vi "FPGA_bubble_SCTL_FIFO.vi"() -> ()   [LabVIEW 2020]
uses:
  <vilib>/Platform/TimedLoop/XDataNode/timing_clust.ctl
  <vilib>/Platform/TimedLoop/XDataNode/nitl_modes.ctl
  <vilib>/Platform/TimedLoop/XDataNode/wakeup.ctl
  <vilib>/rvi/interface/RandomDataEmulation/niFpgaRandomDataHandleErrors.vi
  <vilib>/rvi/Emulation/niFpgaSctlEmulationGetInTimedLoop.vi
  <vilib>/rvi/Emulation/niFpgaEmulationReportErrorSimple.vi
  <vilib>/rvi/Emulation/niFpgaGetClockAttributes.vi
  <vilib>/rvi/Emulation/niFpgaCriticalErrorInLSC.vi
  <vilib>/rvi/DataTransferAndStorage/Container/XNode/niFpgaContainer.xnode
  <vilib>/rvi/interface/RandomDataEmulation/nirviRandomDataFpgaReadWriteTemplate.vi
  <vilib>/platform/TimedLoop/XDataNode/XDataNode.xnode
  <vilib>/Platform/TimedLoop/XDataNode/XDNodeRunTimeDep.lvlib
panel:
  out "sort time (us)":u32
  out "Timed Out? FIFO index":bool
  out "Timed Out? FIFO list":bool
  out "Timed Out FIFO In":bool
  out "Output Valid":bool
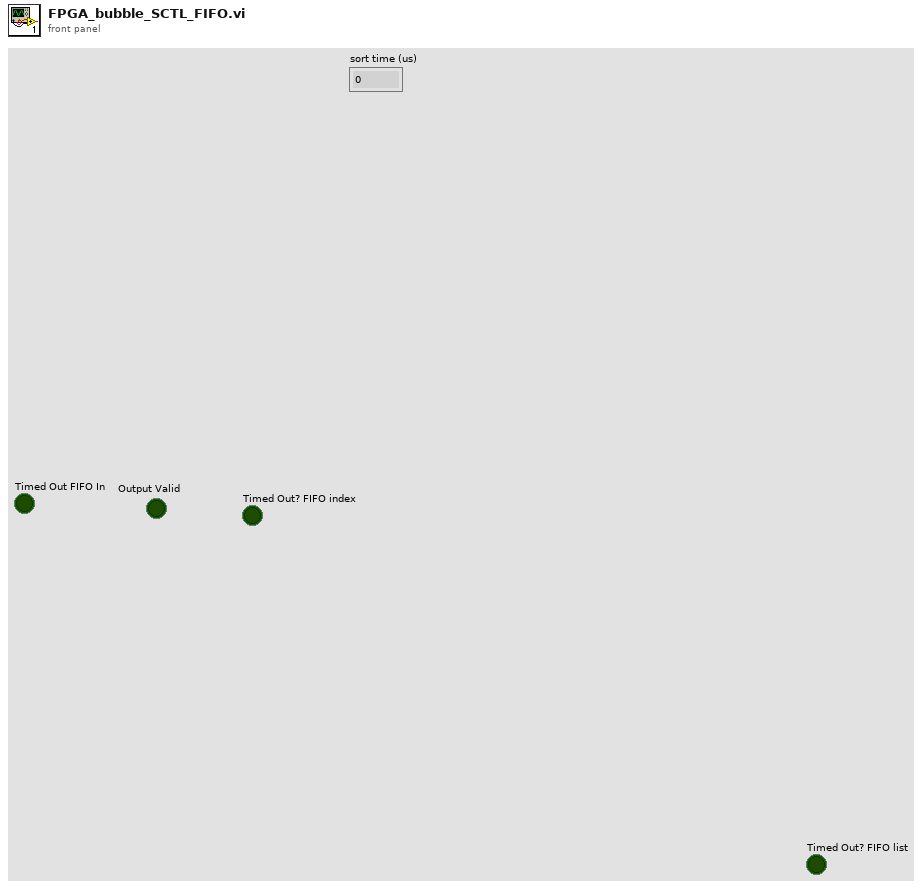
[diagram p1: front panel]
types:
  T1 = typedef "XDNodeRunTimeDep.lvlib/timing_clust.ctl" = cluster{"Expected End [f-1]":u64, "Actual End [f-1]":u64, "Finished Late? [f-1]":bool, "Expected End [i-1]":u64, "Actual End [i-1]":u64, "Finished Late? [i-1]":bool, "Expected Start [i]":u64, "Actual Start [i]":u64, "Expected Start [f]":u64, "Actual Start [f]":u64, "Source Name":string, "Structure Name":string, "Period":i64, "Deadline":i64, "Offset":i64, "Start":i64, "Priority":i32, "Timeout":i32, "Mode":T2, "Wakeup Reason":T3, "Error":errorcluster, "Source Type":string, "Secondary Source Type":string, "Global End Time":u64, "Global Start Time":u64, "Frame Duration":u64, "Iteration Duration":u64, "Assigned CPU":i32, "I/O Scan Engine Mode":u32}
  T2 = typedef "XDNodeRunTimeDep.lvlib/nitl_modes.ctl" = enum32{"No Change", "Process missed periods, maintain original phase", "Discard missed periods, maintain original phase", "Process missed periods, ignore original phase", "Discard missed periods, ignore original phase"}
  T3 = typedef "XDNodeRunTimeDep.lvlib/wakeup.ctl" = enum32{"Normal", "Aborted", "Asynchronous wakeup", "Timing source error", "Timed loop error", "Timeout"}
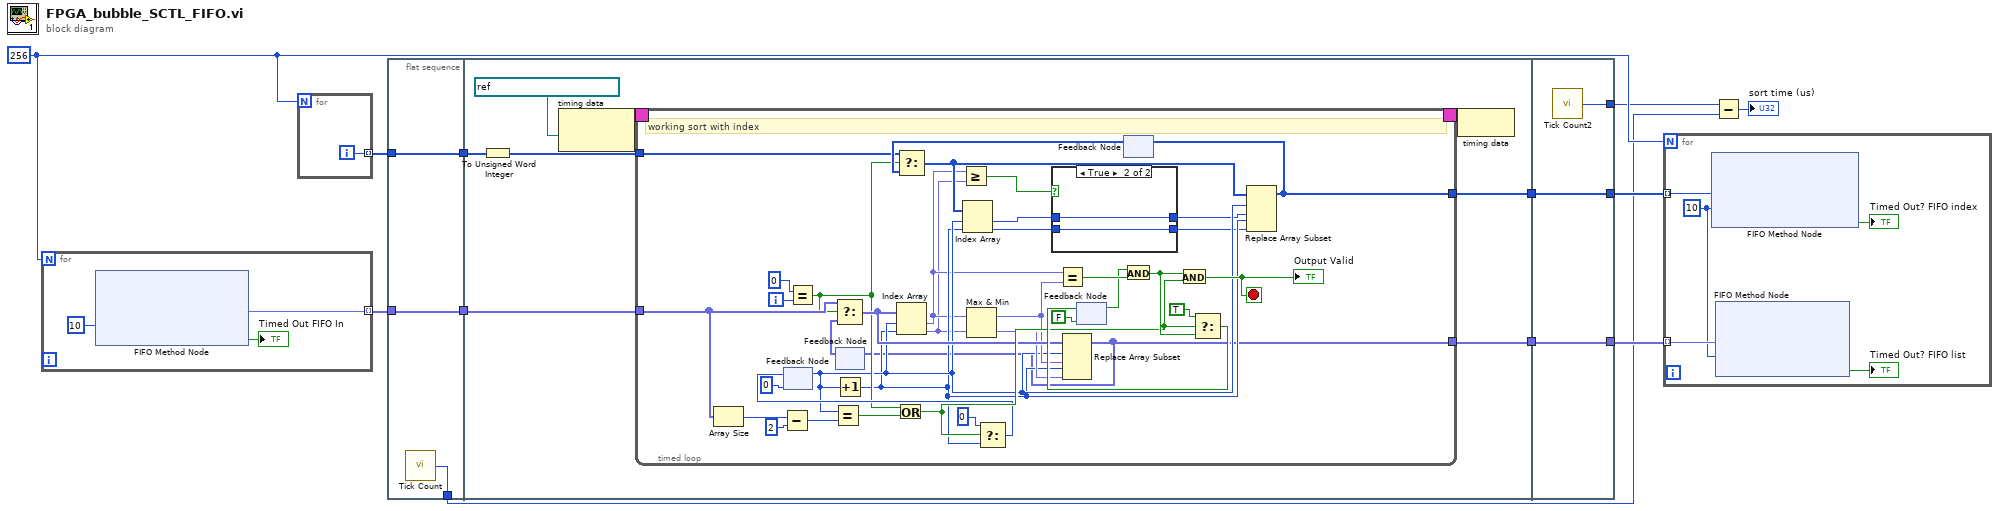
[diagram p0: block diagram]
diagram:
  w9 = 256
  n1 = for {
    N: w9 -> [_]
    tunnel: [w15] -> w11 mode=indexing
    n2 = xnode ("FIFO Method Node")("Timeout"=10) -> ("Element"=w15:fxp<+/-,16,4>, "Timed Out?"=→"Timed Out FIFO In":bool)  [unwired: 1 in, 1 out]
  }
  n3 = for {
    N: w9 -> [_]
    tunnel: [w16] -> w12 mode=indexing
    i -> [w16]
  }
  n4 = flat-sequence {
    tunnel: w11 -> [w18]
    tunnel: w12 -> [w19]
    tunnel: [w19] -> w7
    tunnel: [w18] -> w6
    tunnel: [w17] -> w2
    tunnel: w7 -> [w25]
    tunnel: w6 -> [w22]
    tunnel: [w21] -> w5
    tunnel: [w20] -> w4
    tunnel: [w76] -> w8
    tunnel: [w77] -> w10
    tunnel: w5 -> [w77]
    tunnel: w4 -> [w76]
    tunnel: [w75] -> w3
    frame #0 {
      n5 = call "Tick Count"() -> ("Tick Count(uSec)"=w17:u32)
    }
    frame #1 {
      n6 = To Unsigned Word Integer(number=w25) -> (unsigned 16bit integer=w24:u16[])
      n7 = node-c288(refnum<k21> "40 MHz Onboard Clock" ("Source Name")) -> (w27:T1)
      n8 = timed-loop {
        tunnel: w22 -> [w61]
        tunnel: w24 -> [w40]
        timing: w27 -> [_]
        timing-out: [_] -> w26
        tunnel: [w29] -> w21
        tunnel: [w28] -> w20
        i -> [w44]
        stop <- w45 stop-if-true
        # "working sort with index"
        n9 = Array Size(array=w61) -> (size(s)=w64:i32)
        n10 = Subtract(x=w64, y=2) -> (x-y=w62:i32)
        n11 = feedback #1(0 ("y")) -> (w38:i32)
        n12 = Equal?(x=0, y=w44) -> (x = y?=w39:bool)
        n13 = Equal?(x=w38, y=w62) -> (x = y?=w49:bool)
        n14 = feedback #2() -> (w54:fxp<+/-,16,4>[])  [unwired: 1 in]
        n15 = Select(t=w61, s=w39, f=w54) -> (s? t:f=w48:fxp<+/-,16,4>[])
        n16 = Increment(x=w38) -> (x+1=w37:i32)
        n17 = Or(x=w39, y=w49) -> (x .or. y?=w52:bool)
        n18 = Index Array(array=w48, index #1=w38, index #2=w37) -> (element #1=w32:fxp<+/-,16,4>, element #2=w31:fxp<+/-,16,4>)
        n19 = Greater Or Equal?(x=w32, y=w31) -> (x >= y?=w30:bool)
        n20 = Max & Min(x=w32, y=w31) -> (max(x,y)=w47:fxp<+/-,16,4>, min(x,y)=w46:fxp<+/-,16,4>)
        n21 = Select(t=0 ("y"), s=w52, f=w37) -> (s? t:f=w50:i32)
        n22 = feedback-in #1(w50) -> ()
        n23 = Equal?(x=w32, y=w47) -> (x = y?=w60:bool)
        n24 = Replace Array Subset(array=w48, new element #1=w47, index #1=w38, new element #2=w46, index #2=w37) -> (w29:fxp<+/-,16,4>[])
        n25 = feedback-in #2(w29) -> ()
        n26 = feedback #3(FALSE ("t")) -> (w57:bool)
        n27 = feedback #4() -> (w42:u16[])  [unwired: 1 in]
        n28 = Select(t=w40, s=w39, f=w42) -> (s? t:f=w41:u16[])
        n29 = Index Array(array=w41, index #1=w38, index #2=w37) -> (element #1=w36:u16, element #2=w33:u16)
        n30 = case shown="True" w30 {
          tunnel: w36 -> [w66 w68]
          tunnel: [w65 w68] -> w35
          tunnel: [w66 w67] -> w34
          tunnel: w33 -> [w65 w67]
          frame False {
          }
          frame True {
          }
        }
        n31 = And(x=w57, y=w60) -> (x .and. y?=w55:bool)
        n32 = And(x=w55, y=w52) -> (x .and. y?=w45:bool)
        "Output Valid" <- w45
        n33 = Select(t=TRUE, s=w52, f=w55) -> (s? t:f=w58:bool)
        n34 = feedback-in #3(w58) -> ()
        n35 = Replace Array Subset(array=w41, new element #1=w35, index #1=w38, new element #2=w34, index #2=w37) -> (w28:u16[])
        n36 = feedback-in #4(w28) -> ()
      }
      n37 = node-c288(w26) -> ()
    }
    frame #2 {
      n38 = call "Tick Count2"() -> ("Tick Count(uSec)"=w75:u32)
    }
  }
  n39 = for {
    N: w9 -> [_]
    tunnel: w10 -> [w81] mode=indexing
    tunnel: w8 -> [w80] mode=indexing
    w79 = 10 ("Timeout")
    n40 = xnode ("FIFO Method Node")("Element"=w80, "Timeout"=w79) -> ("Timed Out?"=→"Timed Out? FIFO index":bool)  [unwired: 1 in, 1 out]
    n41 = xnode ("FIFO Method Node")("Element"=w81, "Timeout"=w79) -> ("Timed Out?"=→"Timed Out? FIFO list":bool)  [unwired: 1 in, 1 out]
  }
  n42 = Subtract(x=w3, y=w2) -> (x-y=→"sort time (us)":u32)
